vi "extract From Input Packet Inputs.vi"(11 "instance":i32) -> (3 "function return":u16)   [LabVIEW 2022 SP3, in "SADI_FW3.lvlib"]
doc: "SADI_API_Wrapper uint16_t extractFromInputPacket_Inputs(int instance);"
uses:
  SADI_FW3.lvlib
  SADI_FW3.dll
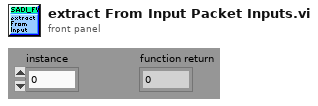
[diagram p1: front panel]
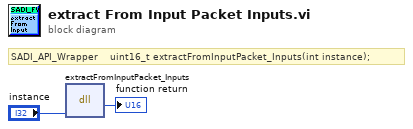
[diagram p0: block diagram]
diagram:
  # "SADI_API_Wrapper    uint16_t extractFromInputPacket_Inputs(int instance);"
  n1 = dll-call lib="C:/Users/scer/OneDrive - University of Florida/eml4314c/eml4314SP23/resources/release_2_3_23/LV/LVLib/SADI_FW3.*" fn="extractFromInputPacket_Inputs"("instance"="instance") -> (→"function return":u16)  [unwired: 4 in, 2 out]
